vi "Get3PhasePhasors.vi"(11 "Group Phasors":T1[](array[typedef])) -> (3 "3-phase Phasors":cdb[](array[numeric]))   [LabVIEW 2017, in "McsaAnalysisLowRate.lvlib"]
uses:
  <vilib>/addons/InsightCM/Devices/Shared/Mcsa/McsaAnalysisLowRate/McsaAnalysisLowRate.lvlib
  <vilib>/addons/InsightCM/Utilities/Analysis/MCSA/controls/McsaChannelPhasor.ctl
  <vilib>/addons/InsightCM/Utilities/Analysis/MCSA/McsaAnalysisFunctions.lvlib
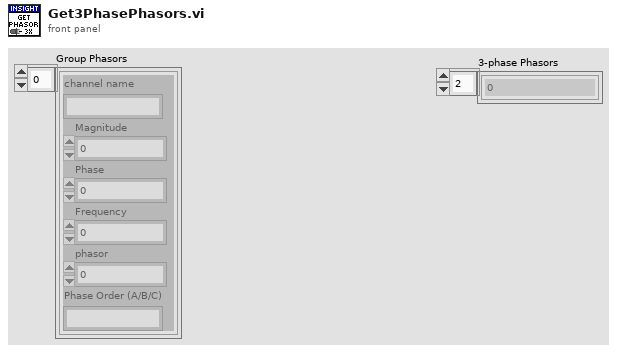
[diagram p1: front panel]
types:
  T1 = typedef "McsaAnalysisFunctions.lvlib/McsaChannelPhasor.ctl" = cluster{"channel name":string, "Magnitude":dbl, "Phase":dbl, "Frequency":dbl, "phasor":cdb, "Phase Order (A/B/C)":string}
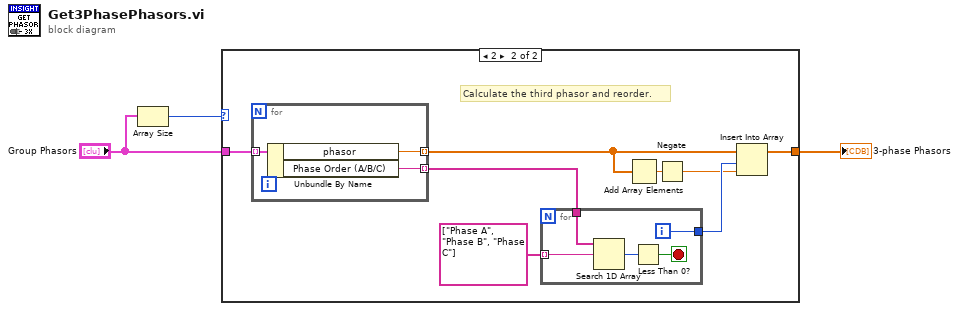
[diagram p0: block diagram]
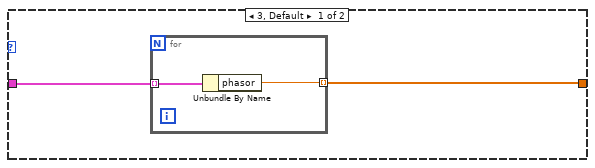
[diagram p2: hidden frame]
diagram:
  n1 = Array Size(array="Group Phasors") -> (size(s)=w1:i32)
  n2 = case shown="2" w1 {
    tunnel: "Group Phasors" -> [w5 w14]
    tunnel: [w4 w11] -> w2
    frame 3, Default {
      n3 = for {
        tunnel: w5 -> [w7] mode=indexing
        tunnel: [w6] -> w4 mode=indexing
        n4 = Unbundle By Name(w7) -> ("phasor"=w6:cdb)
      }
    }
    frame 2 {
      # "Calculate the third phasor and reorder."
      n5 = for {
        tunnel: w14 -> [w23] mode=indexing
        tunnel: [w22] -> w9 mode=indexing
        tunnel: [w21] -> w13 mode=indexing
        n6 = Unbundle By Name(w23) -> ("phasor"=w22:cdb, "Phase Order (A/B/C)"=w21:string)
      }
      n7 = for {
        tunnel: w13 -> [w20]
        tunnel: string[] ["Phase A", "Phase B", "Phase C"] -> [w18] mode=indexing
        tunnel: [w16] -> w12
        i -> [w16]
        stop <- w19 stop-if-true
        n8 = Search 1D Array(1D array=w20, element=w18) -> (index of element=w17:i32)  [unwired: 1 in]
        n9 = Less Than 0?(x=w17) -> (x < 0?=w19:bool)
      }
      n10 = Add Array Elements(numeric array=w9) -> (sum=w10:cdb)
      n11 = Negate(x=w10) -> (-x=w8:cdb)
      n12 = Insert Into Array(array=w9, index=w12, new element=w8) -> (w11:cdb[])
    }
  }
  "3-phase Phasors" <- w2
